vi "task1.vi"() -> (0 "stop":bool=TRUE, 1 "Chart":dbl(graph))   [LabVIEW 2013]
doc: "That.vi is to be used in conjunction with This.vi using VI server. That.vi does run indepently of This.vi. It is necessary to press the Stop button on the front panel of That.vi to halt its execution."
uses:
  <vilib>/Utility/error.llb/DialogType.ctl
  Global 1.vi
panel:
  out "Cycle":i32
  out "Finished":bool
  out "Heartbeat":bool
  out "Time Stamp":timestamp
  in  "error in (no error)":errorcluster
  out "error out":errorcluster
  # "Run the main.vi to programmatically start and stop the task1.vi."
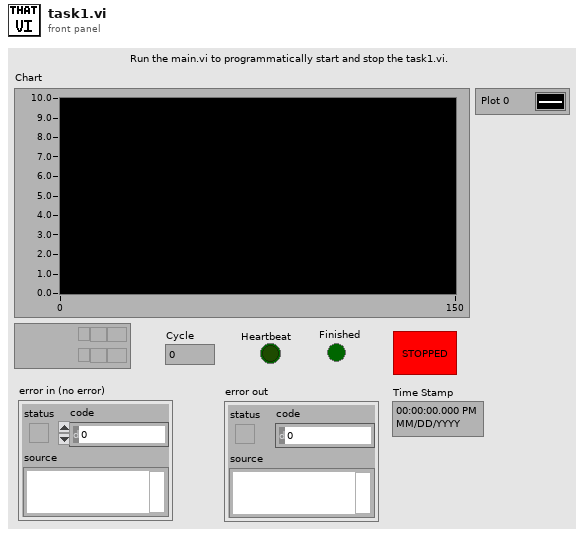
[diagram p1: front panel]
types:
  T1 = typedef "DialogType.ctl" = u16
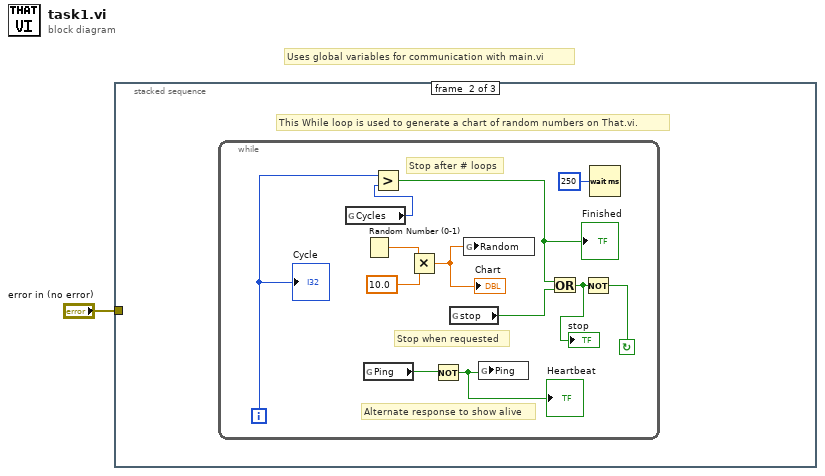
[diagram p0: block diagram]
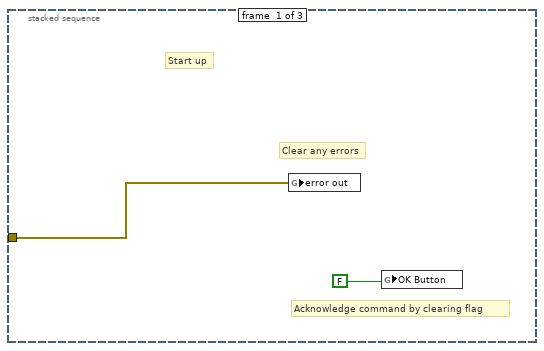
[diagram p2: hidden frame]
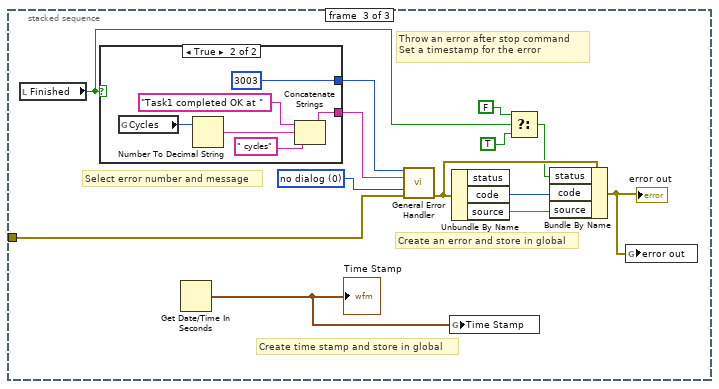
[diagram p3: hidden frame]
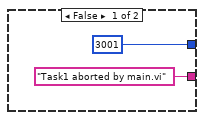
[diagram p4: hidden frame]
diagram:
  # "Uses global variables for communication with main.vi"
  n1 = stacked-sequence {
    tunnel: "error in (no error)" -> [w3 _ w27]
    frame #0 {
      # "Start up"
      # "Acknowledge command by clearing flag"
      # "Clear any errors"
      n2 = global write "Global 1.vi" "error out"(w3) -> ()
      n3 = global write "Global 1.vi" "OK Button"(FALSE) -> ()
    }
    frame #1 {
      # "This While loop is used to generate a chart of random numbers on That.vi."
      n4 = while {
        i -> [w4]
        stop <- w15 continue-if-true
        # "Stop after # loops"
        # "Alternate response to show alive"
        # "Stop when requested"
        n5 = global read "Global 1.vi" "Cycles"() -> (w5:i32)
        n6 = Random Number (0-1)() -> (number: 0 to 1=w14:dbl)
        n7 = global read "Global 1.vi" "Ping"() -> (w10:bool)
        n8 = Greater?(x=w4, y=w5) -> (0:w7:bool)
        "Finished" <- w7
        n9 = Multiply(x=w14, y=10.0) -> (x*y=w11:dbl)
        "Chart" <- w11
        n10 = Not(x=w10) -> (.not. x?=w9:bool)
        "Heartbeat" <- w9
        n11 = global read "Global 1.vi" "stop"() -> (w8:bool)
        n12 = global write "Global 1.vi" "Random"(w11) -> ()
        n13 = global write "Global 1.vi" "Ping"(w9) -> ()
        n14 = Or(x=w7, y=w8) -> (x .or. y?=w6:bool)
        "stop" <- w6
        n15 = Not(x=w6) -> (.not. x?=w15:bool)
        n16 = Wait (ms)(milliseconds to wait=u32 250) -> ()  [unwired: 1 out]
        "Cycle" <- w4
      }
    }
    frame #2 {
      w28 = T1 0 items=["no dialog", "OK message", "continue or stop message", "OK message + warnings", "continue/stop + warnings"] ("type of dialog (OK msg:1)")
      # "Create time stamp and store in global"
      # "Select error number and message"
      # "Throw an error after stop command\nSet a timestamp for the error"
      # "Create an error and store in global"
      n17 = local read "Finished"() -> (w23:bool)
      n18 = case shown="True" w23 {
        tunnel: [3001 ("[error code] (0)") 3003 ("[error code] (0)")] -> w24
        tunnel: ["Task1 aborted by main.vi" ("[error source] (\" \")") w31] -> w25
        frame False {
        }
        frame True {
          n19 = global read "Global 1.vi" "Cycles"() -> (w35:i32)
          n20 = Number To Decimal String(number=w35) -> (decimal integer string=w33:string)  [unwired: 1 in]
          n21 = Concatenate Strings("Task1 completed OK at " ("[error source] (\" \")"), w33, " cycles") -> (w31:string)
        }
      }
      n22 = Get Date/Time In Seconds() -> (seconds since 1Jan1904=w26:timestamp)
      "Time Stamp" <- w26
      n23 = call <vilib>:"General Error Handler.vi"("[error code] (0)"=w24, "[error source] (\" \")"=w25, "type of dialog (OK msg:1)"=w28, "error in (no error)"=w27) -> ("error out"=w18:errorcluster)  [unwired: 7 in, 4 out]
      n24 = global write "Global 1.vi" "Time Stamp"(w26) -> ()
      n25 = Unbundle By Name(w18) -> ("code"=w20:i32, "source"=w19:string)  [unwired: 1 out]
      n26 = Select(t=FALSE, s=w23, f=TRUE) -> (s? t:f=w16:bool)
      n27 = Bundle By Name(cluster=w18, "status"=w16, "code"=w20, "source"=w19) -> (w17:errorcluster)
      "error out" <- w17
      n28 = global write "Global 1.vi" "error out"(w17) -> ()
    }
  }
